vi "VI Tree.vi"   [LabVIEW 2021, in "Keithley 2200 Series.lvlib"]
doc: "This is the instrument driver for the Keithley 2200 Series Programable Power Supplies. The VI Tree displays all the user-callable VIs of the instrument driver in an organized table."
uses:
  <instrlib>/Keithley 2200 Series/Keithley 2200 Series.lvlib
panel:
  # "(c) Copyright 2012 Keithley Instruments Inc  ALL RIGHTS RESERVED."
  # "SEE DIAGRAM\nFOR VI TREE."
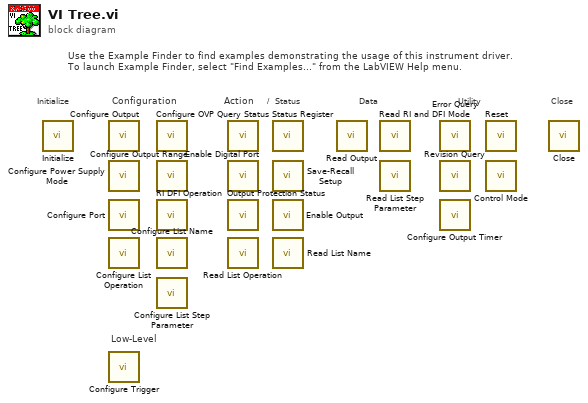
[diagram p0: block diagram]
diagram:
  # "Low-Level"
  # "/"
  # "Action"
  # "Close"
  # "Configuration"
  # "Initialize"
  # "Use the Example Finder to find examples demonstrating the usage of this instrument driver.\nTo launch Example Finder, select \"Find Examples...\" from the LabVIEW Help menu."
  # "Status"
  # "Data"
  # "Utility"
  n1 = call <instrlib>:"Initialize.vi"() -> ()  [unwired: 10 in, 2 out]
  n2 = call <instrlib>:"Configure Output.vi"() -> ()  [unwired: 14 in, 2 out]
  n3 = call <instrlib>:"Configure Power Supply Mode.vi"() -> ()  [unwired: 10 in, 2 out]
  n4 = call <instrlib>:"Configure Port.vi"() -> ()  [unwired: 10 in, 2 out]
  n5 = call <instrlib>:"Configure List Operation.vi"() -> ()  [unwired: 14 in, 2 out]
  n6 = call <instrlib>:"Configure Trigger.vi"() -> ()  [unwired: 10 in, 2 out]
  n7 = call <instrlib>:"Configure OVP.vi"() -> ()  [unwired: 10 in, 2 out]
  n8 = call <instrlib>:"Configure Output Range.vi"() -> ()  [unwired: 14 in, 2 out]
  n9 = call <instrlib>:"RI DFI Operation.vi"() -> ()  [unwired: 10 in, 2 out]
  n10 = call <instrlib>:"Configure List Name.vi"() -> ()  [unwired: 10 in, 2 out]
  n11 = call <instrlib>:"Configure List Step Parameter.vi"() -> ()  [unwired: 10 in, 2 out]
  n12 = call <instrlib>:"Query Status.vi"() -> ()  [unwired: 9 in, 3 out]
  n13 = call <instrlib>:"Enable Digital Port.vi"() -> ()  [unwired: 10 in, 2 out]
  n14 = call <instrlib>:"Output Protection Status.vi"() -> ()  [unwired: 9 in, 3 out]
  n15 = call <instrlib>:"Read List Operation.vi"() -> ()  [unwired: 8 in, 4 out]
  n16 = call <instrlib>:"Status Register.vi"() -> ()  [unwired: 9 in, 3 out]
  n17 = call <instrlib>:"Save-Recall Setup.vi"() -> ()  [unwired: 10 in, 2 out]
  n18 = call <instrlib>:"Enable Output.vi"() -> ()  [unwired: 10 in, 2 out]
  n19 = call <instrlib>:"Read List Name.vi"() -> ()  [unwired: 9 in, 3 out]
  n20 = call <instrlib>:"Read Output.vi"() -> ()  [unwired: 13 in, 3 out]
  n21 = call <instrlib>:"Read RI and DFI Mode.vi"() -> ()  [unwired: 8 in, 4 out]
  n22 = call <instrlib>:"Read List Step Parameter.vi"() -> ()  [unwired: 8 in, 4 out]
  n23 = call <instrlib>:"Error Query.vi"() -> ()  [unwired: 8 in, 4 out]
  n24 = call <instrlib>:"Revision Query.vi"() -> ()  [unwired: 8 in, 4 out]
  n25 = call <instrlib>:"Configure Output Timer.vi"() -> ()  [unwired: 10 in, 2 out]
  n26 = call <instrlib>:"Reset.vi"() -> ()  [unwired: 10 in, 2 out]
  n27 = call <instrlib>:"Control Mode.vi"() -> ()  [unwired: 10 in, 2 out]
  n28 = call <instrlib>:"Close.vi"() -> ()  [unwired: 11 in, 1 out]
